vi "Poll Heaters.vi"(8 "error in (no error)":errorcluster, 11 "cRIO-CO2 in":refnum<class "cRIO-CO2.lvclass">) -> (0 "error out":errorcluster)   [LabVIEW 2015, in "cRIO-Carbondioxide.lvlib" / "cRIO-CO2.lvlib" / "cRIO-CO2.lvclass"]
uses:
  cRIO-CO2.lvclass
  <vilib>/ActorFramework/Actor/Actor.lvclass/Actor.ctl
  <vilib>/ActorFramework/Message Enqueuer/Message Enqueuer.lvclass/Message Enqueuer.ctl
  Blowers Heaters Enumerator.ctl
  cRIO-CO2 Messages/Launch Blower Msg/Launch Blower Msg.lvclass/Launch Blower Msg.ctl
  <vilib>/ActorFramework/Message Enqueuer/Init from Existing Queue.vi
  <vilib>/ActorFramework/Message Enqueuer/Enqueue.vi
  <vilib>/ActorFramework/Message Priority Queue/Priority Enqueue.vi
  <vilib>/ActorFramework/Message Enqueuer/Message Enqueuer.lvclass
  cRIO-CO2 Messages/Launch Piston Heater Msg/Launch Piston Heater Msg.lvclass
  cRIO-CO2 Messages/Launch Blower Msg/Launch Blower Msg.lvclass
  cRIO-CO2 Messages/Launch Syringe Heater Msg/Launch Syringe Heater Msg.lvclass
  <vilib>/ActorFramework/Actor/Actor.lvclass
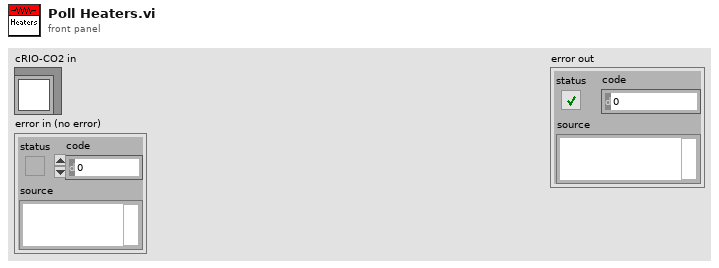
[diagram p1: front panel]
types:
  T1 = typedef "cRIO-Carbondioxide.lvlib/cRIO-CO2.lvlib/cRIO-CO2.lvclass/Blowers Heaters Enumerator.ctl" = enum16{"Tank Blower 1", "Tank Blower 2", "Tank Blower 3", "Tank Blower 4", "Syringe Blower", "Syringe Heater", "Piston Heater", "Undefined"}
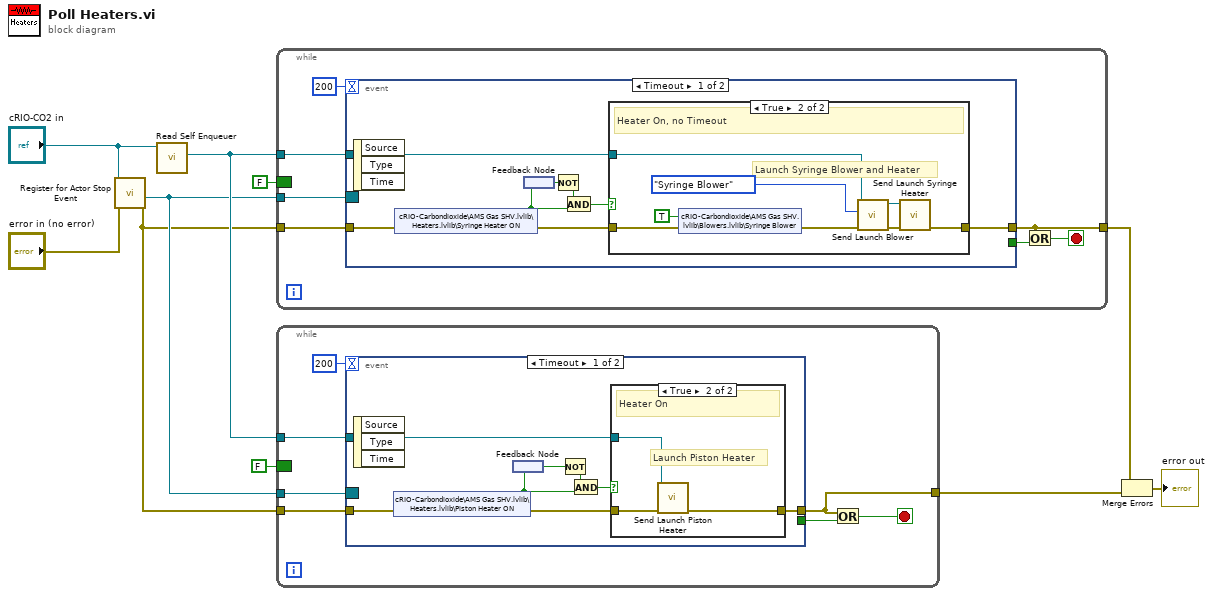
[diagram p0: block diagram]
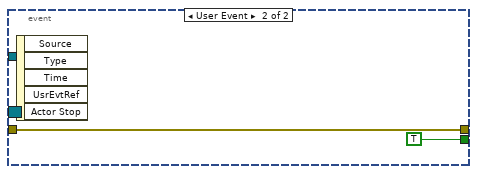
[diagram p3: hidden frame]
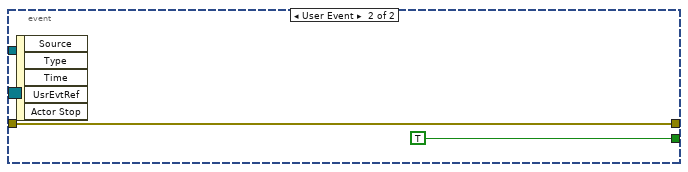
[diagram p5: hidden frame]
diagram:
  n1 = call "Register for Actor Stop Event.vi"("error in (no error)"="error in (no error)", "cRIO-CO2 in"="cRIO-CO2 in") -> ("error out"=w4:errorcluster, "Event Registration Refnum"=w5:refnum<event-registration>)  [unwired: 7 in, 1 out]
  n2 = call <vilib>:"Read Self Enqueuer.vi"("Actor"="cRIO-CO2 in") -> ("Self Enqueuer"=w6:refnum<class "Message Enqueuer.lvclass">)  [unwired: 10 in]
  n3 = while {
    tunnel: w6 -> [w17]
    border: FALSE ("Boolean") -> [_]
    tunnel: w4 -> [w16]
    tunnel: w5 -> [w13]
    tunnel: [w11] -> w2
    stop <- w14 stop-if-true
    n4 = event shown="[0] Timeout" {
      selector: w13 -> [_ _]
      dyn-events: _ -> [_ _]
      timeout: 200 -> [_ _]
      tunnel: [w25 w34] -> w11
      tunnel: w17 -> [w23 _]
      tunnel: w16 -> [w18 w34]
      tunnel: [_ TRUE] -> w12
      event Timeout {
        n5 = event-data() -> ()  [unwired: 1 in, 3 out]
        n6 = shared-variable "cRIO-Carbondioxide\\AMS Gas SHV.lvlib\\Heaters.lvlib\\Syringe Heater ON"(error in=w18) -> (w19:bool, error out=w24:errorcluster)
        n7 = feedback #1() -> (w21:bool)
        n8 = feedback-in #1(w19) -> ()
        n9 = Not(x=w21) -> (.not. x?=w20:bool)
        n10 = And(x=w20, y=w19) -> (x .and. y?=w22:bool)
        n11 = case shown="True" w22 {
          tunnel: w23 -> [_ w31]
          tunnel: [_ w33] -> w25
          tunnel: w24 -> [_ w29]
          frame False {
          }
          frame True {
            # "Launch Syringe Blower and Heater"
            # "Heater On, no Timeout"
            n12 = shared-variable "cRIO-Carbondioxide\\AMS Gas SHV.lvlib\\Blowers.lvlib\\Syringe Blower"(TRUE ("Syringe Blower"), error in=w29) -> (error out=w28:errorcluster)
            n13 = call "Send Launch Blower.vi"("error in (no error)"=w28, "Blower"=Blowers_Heaters_Enumerator."Syringe Blower", "Message Enqueuer"=w31) -> ("error out"=w32:errorcluster, "Message Enqueuer out"=w30:refnum<class "Message Enqueuer.lvclass">)  [unwired: 7 in]
            n14 = call "Send Launch Syringe Heater.vi"("error in (no error)"=w32, "Message Enqueuer"=w30) -> ("error out"=w33:errorcluster)  [unwired: 8 in, 1 out]
          }
        }
      }
      event User Event {
        n15 = event-data() -> ()  [unwired: 1 in, 5 out]
      }
    }
    n16 = Or(x=w11, y=w12) -> (x .or. y?=w14:bool)
  }
  n17 = while {
    tunnel: w6 -> [w42]
    border: FALSE ("Boolean") -> [_]
    tunnel: w5 -> [w38]
    tunnel: w4 -> [w41]
    tunnel: [w36] -> w3
    stop <- w39 stop-if-true
    n18 = event shown="[0] Timeout" {
      selector: w38 -> [_ _]
      dyn-events: _ -> [_ _]
      timeout: 200 -> [_ _]
      tunnel: [w50 w54] -> w36
      tunnel: w42 -> [w47 _]
      tunnel: w41 -> [w43 w54]
      tunnel: [_ TRUE] -> w37
      event Timeout {
        n19 = event-data() -> ()  [unwired: 1 in, 3 out]
        n20 = shared-variable "cRIO-Carbondioxide\\AMS Gas SHV.lvlib\\Heaters.lvlib\\Piston Heater ON"(error in=w43) -> (w46:bool, error out=w49:errorcluster)
        n21 = feedback #2() -> (w45:bool)
        n22 = feedback-in #2(w46) -> ()
        n23 = Not(x=w45) -> (.not. x?=w44:bool)
        n24 = And(x=w44, y=w46) -> (x .and. y?=w48:bool)
        n25 = case shown="True" w48 {
          tunnel: w47 -> [_ w51]
          tunnel: [_ w53] -> w50
          tunnel: w49 -> [_ w52]
          frame False {
          }
          frame True {
            # "Launch Piston Heater"
            # "Heater On"
            n26 = call "Send Launch Piston Heater.vi"("error in (no error)"=w52, "Message Enqueuer"=w51) -> ("error out"=w53:errorcluster)  [unwired: 8 in, 1 out]
          }
        }
      }
      event User Event {
        n27 = event-data() -> ()  [unwired: 1 in, 5 out]
      }
    }
    n28 = Or(x=w36, y=w37) -> (x .or. y?=w39:bool)
  }
  n29 = Merge Errors(w2, w3) -> (→"error out":errorcluster)
